vi "Custom_NOR.vi"(9 "Input B":bool, 11 "Input A":bool) -> (3 "Output Y":bool)   [LabVIEW 2026]
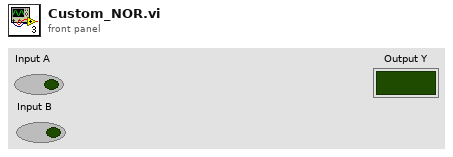
[diagram p1: front panel]
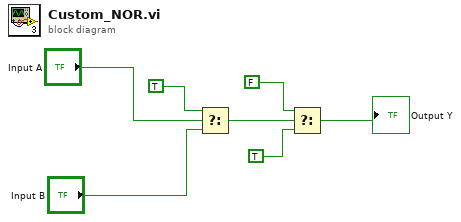
[diagram p0: block diagram]
diagram:
  n1 = Select(t=TRUE, s="Input A", f="Input B") -> (s? t:f=w2:bool)
  n2 = Select(t=FALSE, s=w2, f=TRUE) -> (s? t:f=→"Output Y":bool)
